vi "AnalysisPluginTemplate.vi"(9 "DeviceModel":T7, 10 "PluginInfo":T1, 11 "tdms file in":refnum<k34>) -> (0 "error out":errorcluster, 2 "Messages":T5[](array[typedef]), 3 "tdms file out":refnum<k34>)   [LabVIEW 2017]
uses:
  <vilib>/addons/InsightCM/MessageBus/Base/controls/DeviceModel.ctl
  <vilib>/addons/InsightCM/MessageBus/Base/controls/Device.ctl
  <vilib>/addons/InsightCM/MessageBus/Base/controls/KeyValuePair.ctl
  <vilib>/addons/InsightCM/MessageBus/Base/controls/DeviceState.ctl
  <vilib>/addons/InsightCM/MessageBus/Base/controls/DataGroup.ctl
  <vilib>/addons/InsightCM/MessageBus/Base/controls/BurstModeTrigger.ctl
  <vilib>/addons/InsightCM/MessageBus/Base/controls/Trigger.ctl
  <vilib>/addons/InsightCM/MessageBus/Base/controls/Condition.ctl
  <vilib>/addons/InsightCM/MessageBus/Base/controls/Channel.ctl
  <vilib>/addons/InsightCM/MessageBus/Base/controls/Tag.ctl
  <vilib>/addons/InsightCM/MessageBus/Base/controls/Message.ctl
  <vilib>/addons/InsightCM/MessageBus/Base/controls/MessageHeader.ctl
  <vilib>/addons/InsightCM/Utilities/Misc/controls/AnalysisPluginInfo.ctl
  <vilib>/addons/InsightCM/MessageBus/Base/controls/Metric.ctl
  <vilib>/addons/InsightCM/MessageBus/Base/controls/MetricDefinitionInstance.ctl
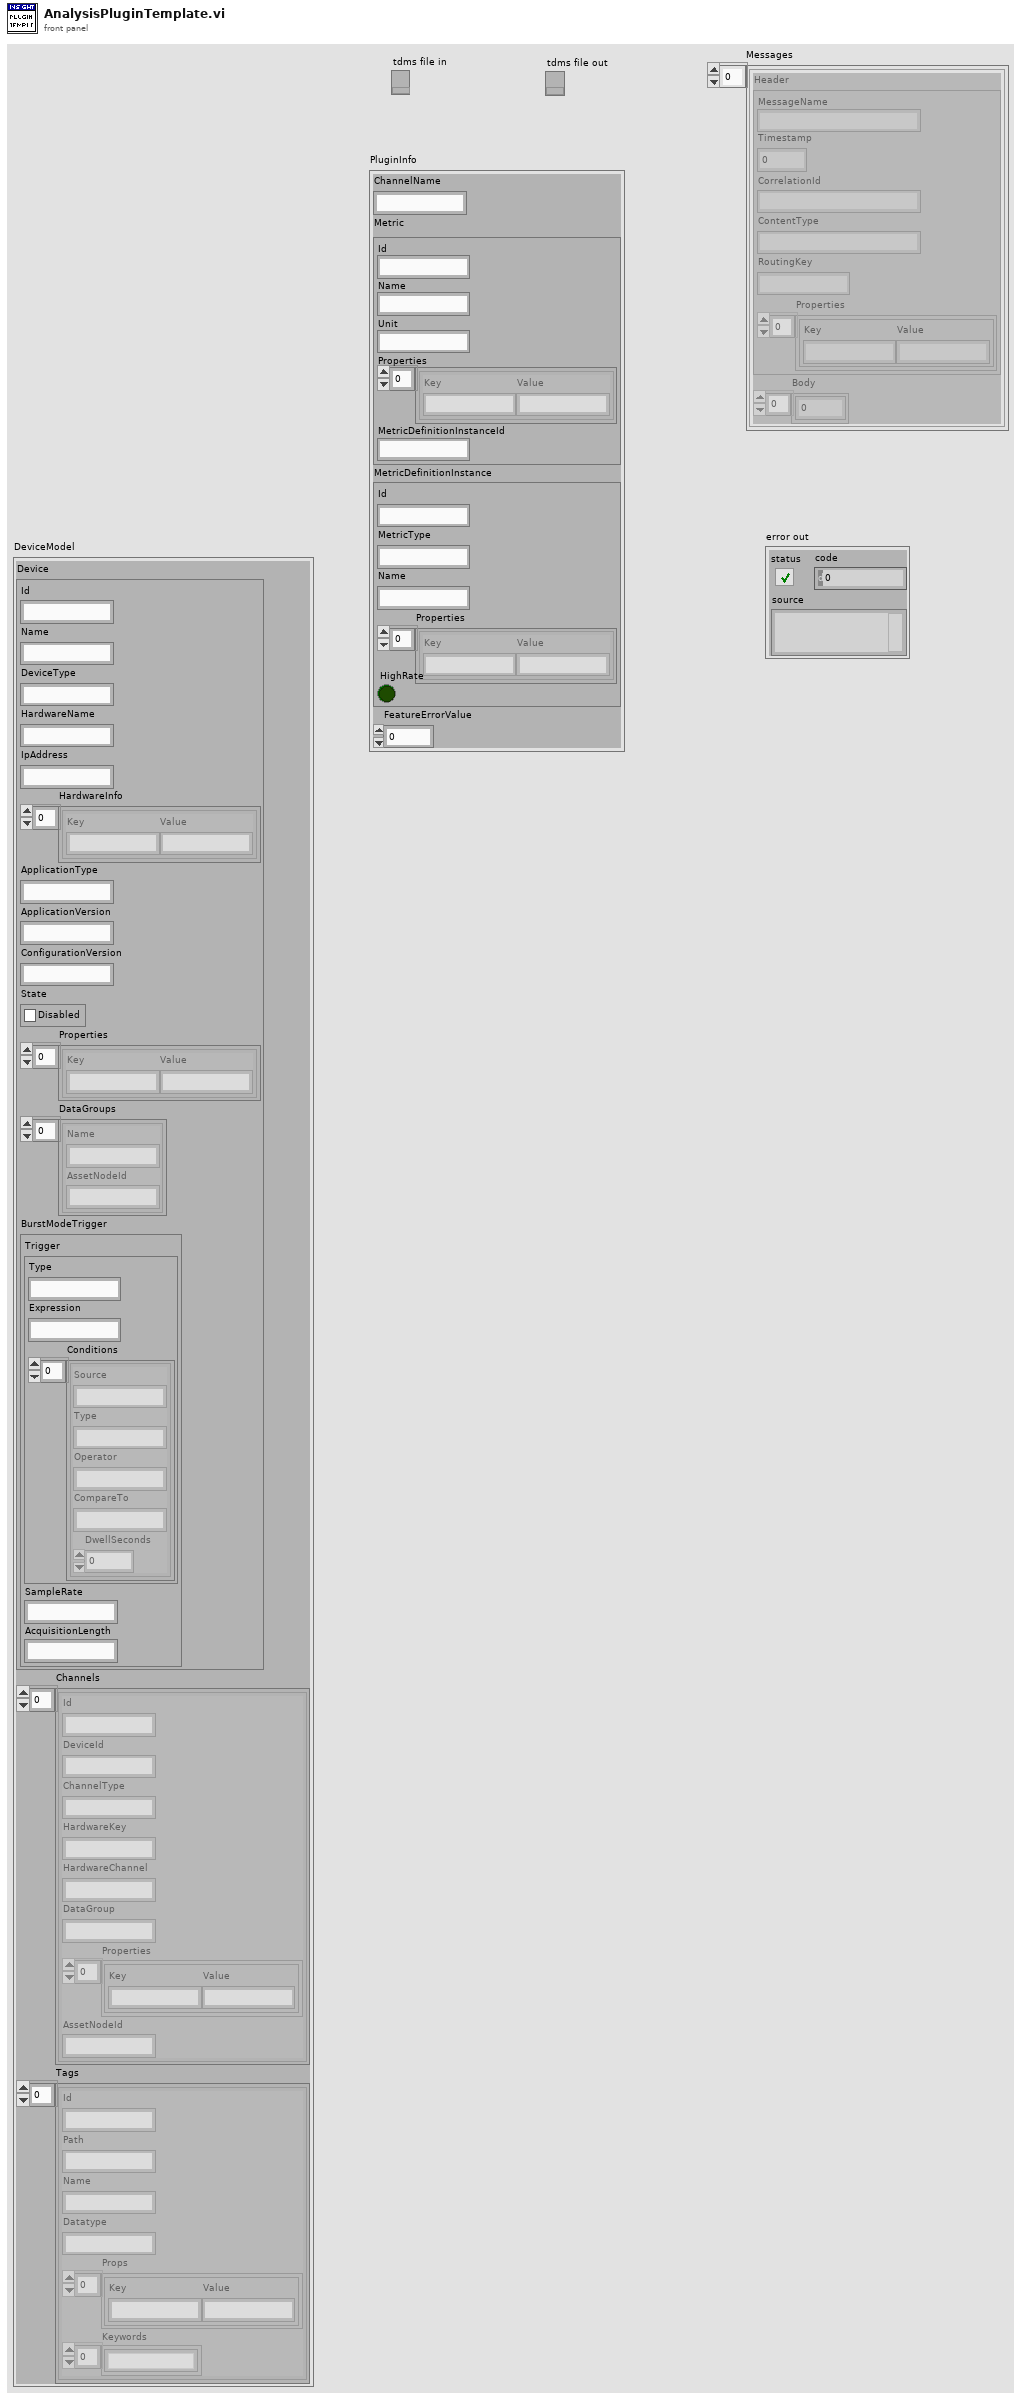
[diagram p1: front panel]
types:
  T1 = typedef "AnalysisPluginInfo.ctl" = cluster{"ChannelName":string, "Metric":T2, "MetricDefinitionInstance":T4, "FeatureErrorValue":dbl}
  T2 = typedef "Metric.ctl" = cluster{"Id":string, "Name":string, "Unit":string, "Properties":T3[], "MetricDefinitionInstanceId":string}
  T3 = typedef "KeyValuePair.ctl" = cluster{"Key":string, "Value":string}
  T4 = typedef "MetricDefinitionInstance.ctl" = cluster{"Id":string, "MetricType":string, "Name":string, "Properties":T3[], "HighRate":bool}
  T5 = typedef "Message.ctl" = cluster{"Header":T6, "Body":u8[]}
  T6 = typedef "MessageHeader.ctl" = cluster{"MessageName":string, "Timestamp":i64, "CorrelationId":string, "ContentType":string, "RoutingKey":string, "Properties":T3[]}
  T7 = typedef "DeviceModel.ctl" = cluster{"Device":T8, "Channels":T14[], "Tags":T15[]}
  T8 = typedef "Device.ctl" = cluster{"Id":string, "Name":string, "DeviceType":string, "HardwareName":string, "IpAddress":string, "HardwareInfo":T3[], "ApplicationType":string, "ApplicationVersion":string, "ConfigurationVersion":string, "State":T9, "Properties":T3[], "DataGroups":T10[], "BurstModeTrigger":T11}
  T9 = typedef "DeviceState.ctl" = cluster{"Disabled":bool}
  T10 = typedef "DataGroup.ctl" = cluster{"Name":string, "AssetNodeId":string}
  T11 = typedef "BurstModeTrigger.ctl" = cluster{"Trigger":T12, "SampleRate":string, "AcquisitionLength":string}
  T12 = typedef "Trigger.ctl" = cluster{"Type":string, "Expression":string, "Conditions":T13[]}
  T13 = typedef "Condition.ctl" = cluster{"Source":string, "Type":string, "Operator":string, "CompareTo":string, "DwellSeconds":dbl}
  T14 = typedef "Channel.ctl" = cluster{"Id":string, "DeviceId":string, "ChannelType":string, "HardwareKey":string, "HardwareChannel":string, "DataGroup":string, "Properties":T3[], "AssetNodeId":string}
  T15 = typedef "Tag.ctl" = cluster{"Id":string, "Path":string, "Name":string, "Datatype":string, "Props":T3[], "Keywords":string[]}
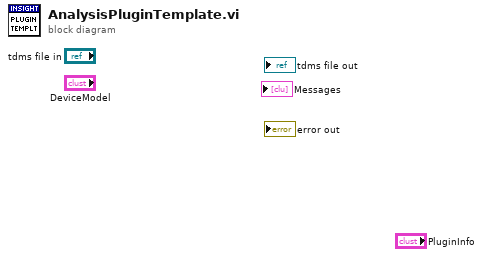
[diagram p0: block diagram]
diagram:
